vi "continuo.vi"() -> ()   [LabVIEW 2016]
uses:
  <vilib>/Utility/file.llb/Write Delimited Spreadsheet (DBL).vi
panel:
  out "division":cluster{dbl[], dbl[]}(graph)
  in  "guardar":bool
  in  "Nombre (guardar como .txt)":path=path "C:/Users/parra/Documents/moke/hj5.txt"
  in  "Lecturas":i32=1
  in  "fin":bool
  out "multimetro":cluster{dbl[], dbl[]}(graph)
  out "lockin":cluster{dbl[], dbl[]}(graph)
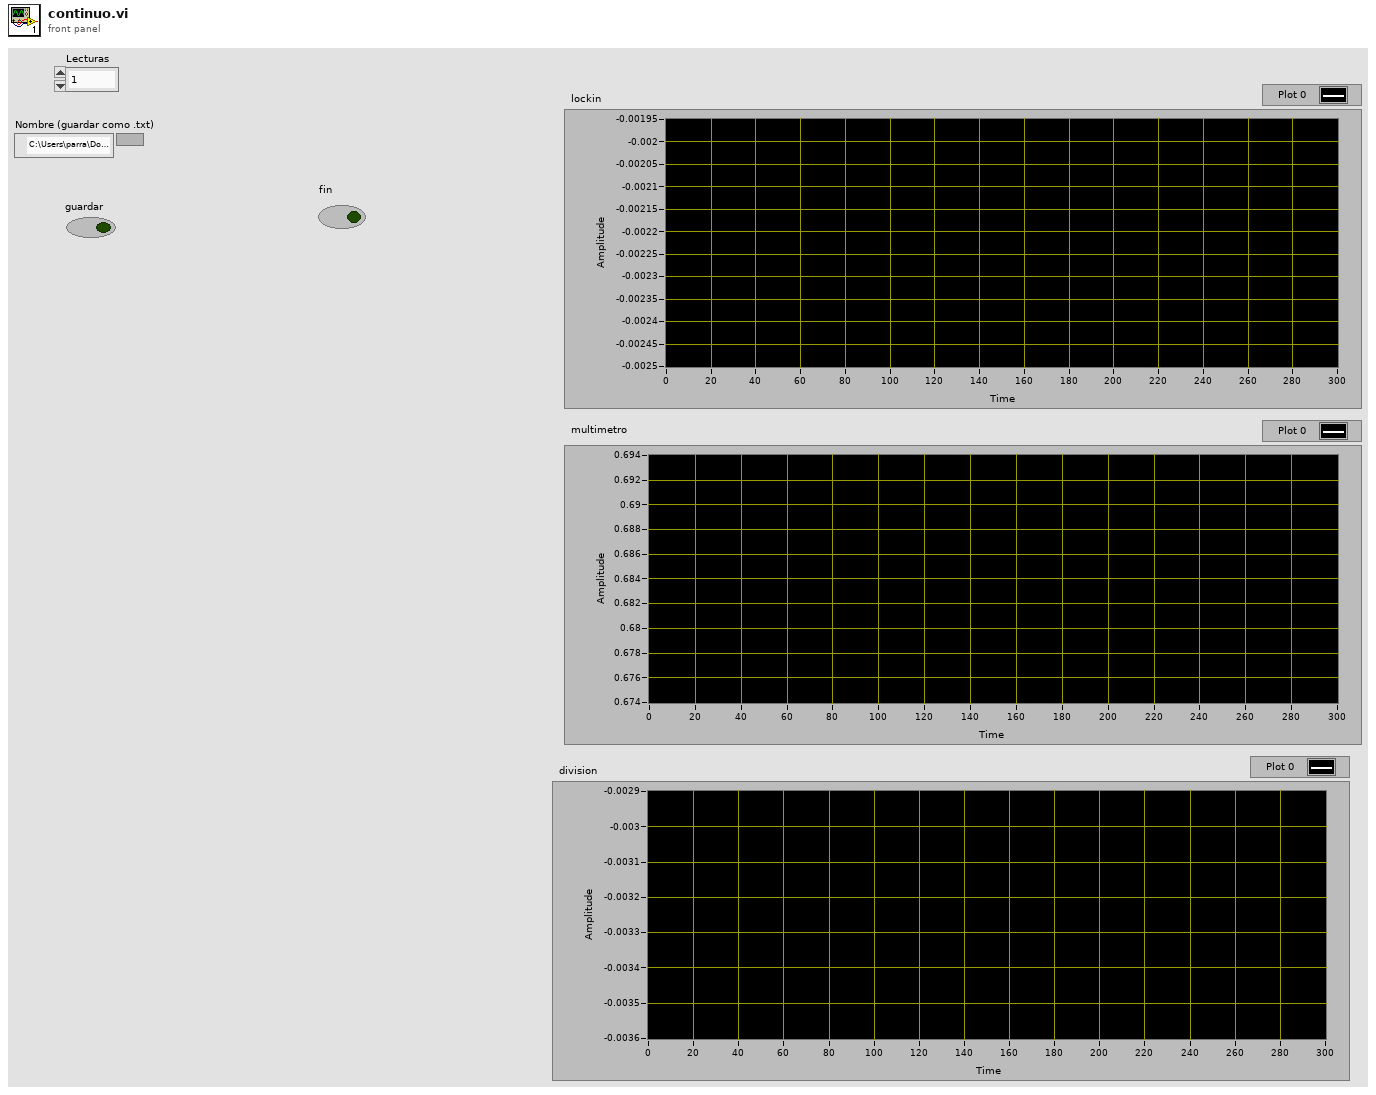
[diagram p1: front panel]
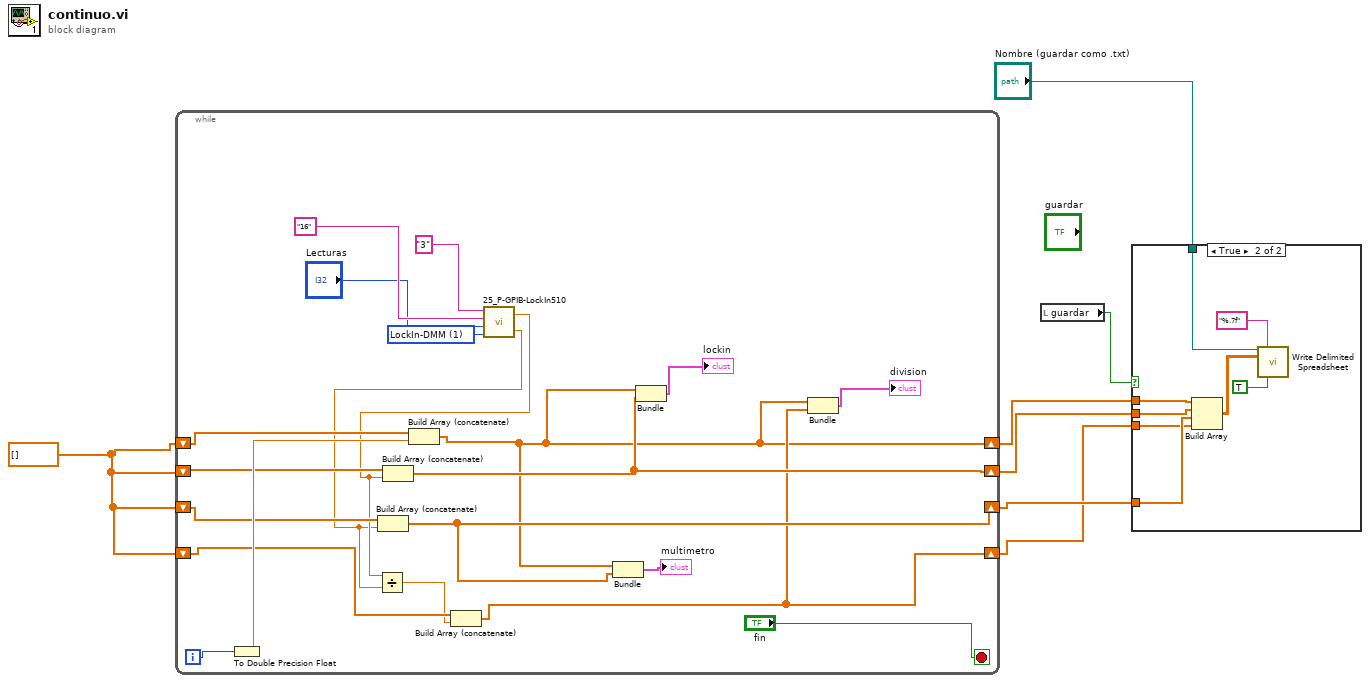
[diagram p0: block diagram]
diagram:
  w2 = dbl[] []
  n1 = while {
    shift-right: [w8] -> w6
    shift-left: w2 -> [w22]
    shift-right: [w16] -> w5
    shift-left: w2 -> [w20]
    shift-right: [w17] -> w4
    shift-left: w2 -> [w19]
    shift-right: [w9] -> w1
    shift-left: w2 -> [w14]
    i -> [w23]
    stop <- "fin" stop-if-true
    w24 = u16 1 items=["LockIn", "LockIn-DMM"] ("Tipo")
    n2 = To Double Precision Float(number=w23) -> (double precision float=w21:dbl)
    n3 = Build Array (concatenate)(w22, w21) -> (w8:dbl[])
    n4 = call "25_P-GPIB-LockIn510.vi"("Tipo"=w24, "Lecturas"="Lecturas", "P-DMM"="16", "P-LockIn"="3") -> ("DMM"=w11:dbl, "LockIn"=w12:dbl)
    n5 = Divide(x=w12, y=w11) -> (x/y=w13:dbl)
    n6 = Build Array (concatenate)(w19, w11) -> (w17:dbl[])
    n7 = Build Array (concatenate)(w20, w12) -> (w16:dbl[])
    n8 = Build Array (concatenate)(w14, w13) -> (w9:dbl[])
    n9 = Bundle(w8, w17) -> (→"multimetro":cluster{dbl[], dbl[]})  [unwired: 1 in]
    n10 = Bundle(w8, w16) -> (→"lockin":cluster{dbl[], dbl[]})  [unwired: 1 in]
    n11 = Bundle(w8, w9) -> (→"division":cluster{dbl[], dbl[]})  [unwired: 1 in]
  }
  n12 = local read "guardar"() -> (w3:bool)
  n13 = case shown="True" w3 {
    tunnel: "Nombre (guardar como .txt)" -> [_ w36]
    tunnel: w6 -> [_ w35]
    tunnel: w5 -> [_ w34]
    tunnel: w4 -> [_ w33]
    tunnel: w1 -> [_ w29]
    frame False {
    }
    frame True {
      n14 = Build Array(w35, w34, w33, w29) -> (w32:dbl[][])
      n15 = call-poly <vilib>:"Write Delimited Spreadsheet.vi"("file path (dialog if empty)"=w36, "format (%.3f)"="%.7f", "2D data"=w32, "transpose? (no:F)"=TRUE) -> ()  [unwired: 10 in, 2 out]
    }
  }
